vi "Unibot - State Machine Controller.vi"(5 "Up Optimal Gain":dbl[](array[numeric])=[-16.4615, -16.2422, -3.1287, -2.0658], 6 "PD Gains":T1={"Kp Up"=14.2, "Kd Up"=1.1, "Kp Down"=15.0, "Kd Down"=0.9}, 7 "Setpoint Theta":dbl(knob) scale=-0.1..0.1, 8 "Enable":bool, 9 "Kill":bool, 11 "States":dbl[](array[numeric])=[-0.0012566370614359172, -0.8117875416876026, 0.0, 0.0]) -> (0 "Status":string="Kill", 2 "Control Effort":dbl=-0.1425196371146851)   [LabVIEW 2012]
uses:
  Unibot - States.ctl
  <vilib>/addons/Control Design/_Implementation/CD State Feedback Controller (Single Output).vi
  <vilib>/addons/Control Design/_Implementation/NI_CD_Implementation.lvlib
panel:
  in  "Setpoint V":dbl(knob) scale=-0.1..0.1
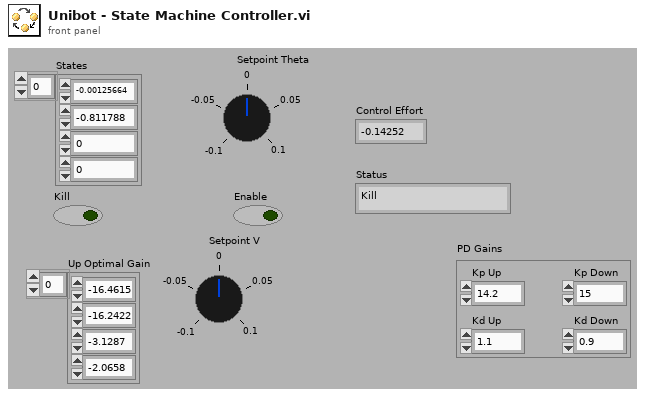
[diagram p1: front panel]
types:
  T1 = cluster{"Kp Up":dbl, "Kd Up":dbl, "Kp Down":dbl, "Kd Down":dbl}
  T2 = typedef "Unibot - States.ctl" = enum16{"Idle", "Balance", "Emergency"}
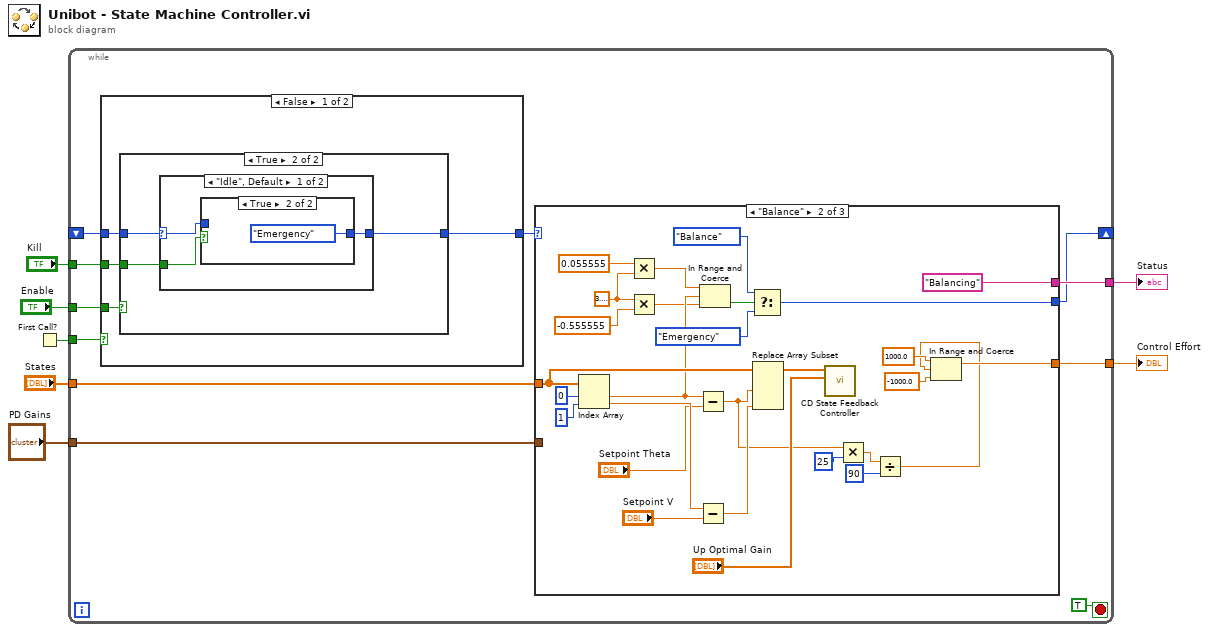
[diagram p0: block diagram]
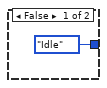
[diagram p2: hidden frame]
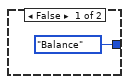
[diagram p3: hidden frame]
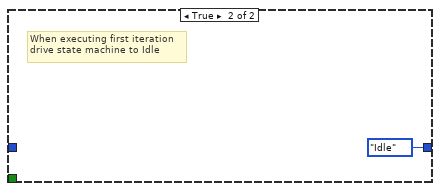
[diagram p5: hidden frame]
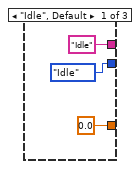
[diagram p6: hidden frame]
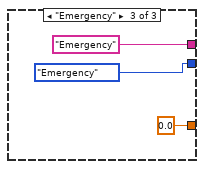
[diagram p7: hidden frame]
diagram:
  n1 = First Call?() -> (First Call?: T/F=w3:bool)
  n2 = while {
    tunnel: "States" -> [w17]
    tunnel: [w13] -> w6
    shift-right: [w12] -> _
    shift-left: _ -> [w14]
    tunnel: [w16] -> w5
    tunnel: "Kill" -> [w15]
    tunnel: w3 -> [w10]
    tunnel: "Enable" -> [w9]
    tunnel: "PD Gains" -> [w8]
    stop <- TRUE stop-if-true
    n3 = case shown="False" w10 {
      tunnel: w15 -> [w22 _]
      tunnel: w14 -> [w21 _]
      tunnel: [w20 Unibot_-_States."Idle" ("Enum")] -> w11
      tunnel: w9 -> [w19 _]
      frame False {
        n4 = case shown="True" w19 {
          tunnel: w22 -> [_ w26]
          tunnel: [Unibot_-_States."Idle" ("Enum") w25] -> w20
          tunnel: w21 -> [_ w24]
          frame False {
          }
          frame True {
            n5 = case shown="\"Idle\", Default" w24 {
              selector: w24 -> [w28 w32]
              tunnel: w26 -> [w29 _]
              tunnel: [w27 w32] -> w25
              frame "Idle", Default {
                n6 = case shown="True" w29 {
                  tunnel: [Unibot_-_States."Balance" ("Enum") Unibot_-_States."Emergency" ("Enum")] -> w27
                  tunnel: w28 -> [_ _]
                  frame False {
                  }
                  frame True {
                  }
                }
              }
              frame "Emergency" {
              }
            }
          }
        }
      }
      frame True {
        # "When executing first iteration\ndrive state machine to Idle"
      }
    }
    n7 = case shown="\"Balance\"" w11 {
      tunnel: w17 -> [_ w58 _]
      tunnel: [0.0 w53 0.0] -> w13
      tunnel: [Unibot_-_States."Idle" ("Enum") w64 Unibot_-_States."Emergency" ("Enum")] -> w12
      tunnel: ["Idle" "Balancing" "Emergency"] -> w16
      tunnel: w8 -> [_ _ _]
      frame "Idle", Default {
      }
      frame "Balance" {
        w51 = 3.141592653589793 ("Setpoint")
        n8 = Index Array(array=w58, index #1=0 ("index"), index #2=1 ("index")) -> (element #1=w57:dbl, element #2=w60:dbl)
        n9 = Multiply(x=0.055555, y=w51) -> (x*y=w49:dbl)
        n10 = Multiply(x=w51, y=-0.555555) -> (x*y=w47:dbl)
        n11 = Subtract(x=w57, y="Setpoint Theta") -> (x-y=w38:dbl)
        n12 = Subtract(x=w60, y="Setpoint V") -> (x-y=w59:dbl)
        n13 = In Range and Coerce(upper limit=w49, x=w57, lower limit=w47) -> (In Range?=w46:bool)  [unwired: 1 out]
        n14 = Select(t=Unibot_-_States."Balance" ("Enum"), s=w46, f=Unibot_-_States."Emergency" ("Enum")) -> (s? t:f=w64:T2)
        n15 = Replace Array Subset(array=w58, new element #1=w38, new element #2=w59) -> (w63:dbl[])  [unwired: 2 in]
        n16 = call-poly <vilib>:"CD State Feedback Controller.vi"("Controller Gain"="Up Optimal Gain", "States"=w63) -> ()  [unwired: 1 in, 9 out]
        n17 = Multiply(x=w38, y=25) -> (x*y=w41:dbl)
        n18 = Divide(x=w41, y=90) -> (x/y=w37:dbl)
        n19 = In Range and Coerce(upper limit=1000.0, x=w37, lower limit=-1000.0) -> (coerced(x)=w53:dbl)  [unwired: 1 out]
      }
      frame "Emergency" {
      }
    }
  }
  "Control Effort" <- w6
  "Status" <- w5
